vi "Advanced Cut - Snippet to Text.vi"(8 "error in (no error)":errorcluster, 11 "Numeric Snippets":dbl[][](array[numeric])) -> (0 "error out":errorcluster, 3 "String Snippets":string[][](array[string]))   [LabVIEW 2016]
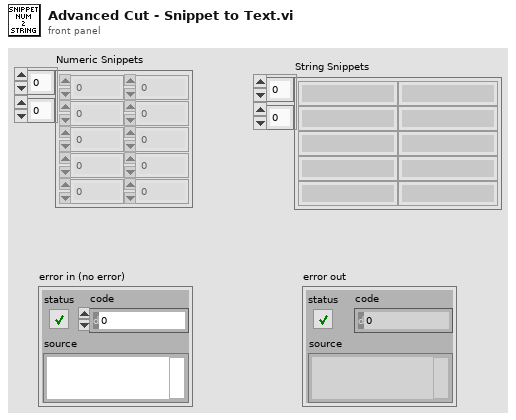
[diagram p1: front panel]
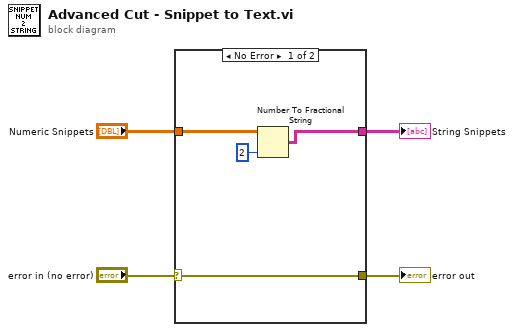
[diagram p0: block diagram]
diagram:
  n1 = case shown="No Error" "error in (no error)" {
    selector: "error in (no error)" -> [w7 w9]
    tunnel: [w7 w9] -> w3
    tunnel: "Numeric Snippets" -> [w6 _]
    tunnel: [w5 _] -> w1
    frame No Error {
      n2 = Number To Fractional String(number=w6, precision (6)=i16 2) -> (F-format string=w5:string[][])  [unwired: 2 in]
    }
    frame Error {
    }
  }
  "error out" <- w3
  "String Snippets" <- w1
